vi "PSConverter.vi"(1 "Current States 2":string[][](table), 2 "PROC":string[](array[string]), 3 "STATES":string[][](array[string]), 4 "Input claster":cluster{u32, u8}[](array[cluster])) -> (0 "Current States":string[][](table))   [LabVIEW 2010]
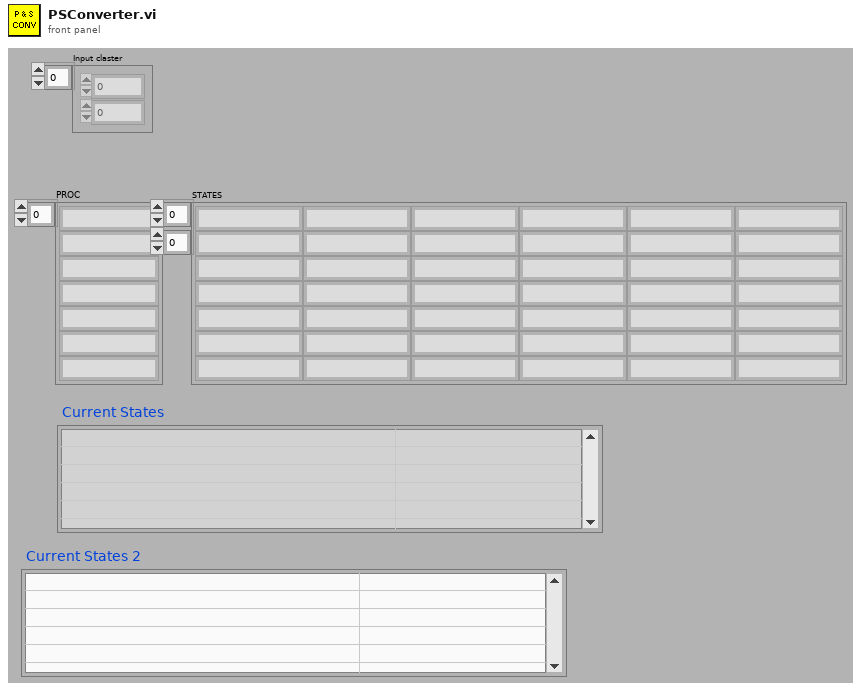
[diagram p1: front panel]
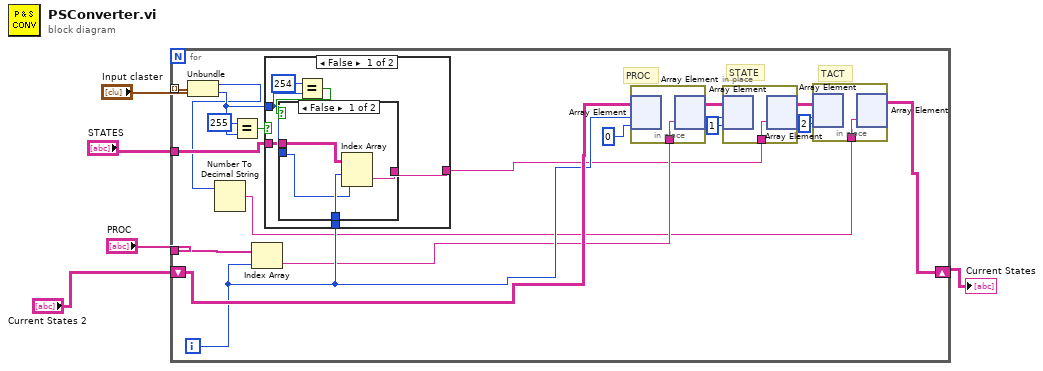
[diagram p0: block diagram]
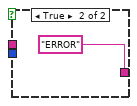
[diagram p2: hidden frame]
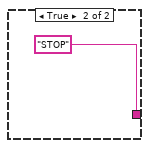
[diagram p3: hidden frame]
diagram:
  n1 = for {
    tunnel: "Input claster" -> [w25] mode=indexing
    tunnel: "PROC" -> [w21]
    tunnel: "STATES" -> [w20]
    shift-right: [w6] -> w5
    shift-left: "Current States 2" -> [w18]
    i -> [w17]
    # "TACT"
    # "STATE"
    # "PROC"
    n2 = Unbundle(w25) -> (w19:u32, w22:u8)
    n3 = Number To Decimal String(number=w19) -> (decimal integer string=w7:string)  [unwired: 1 in]
    n4 = Equal?(x=u8 255, y=w22) -> (x = y?=w23:bool)
    n5 = Index Array(array=w21, index=w17) -> (element=w15:string)
    n6 = case shown="False" w23 {
      tunnel: w22 -> [w31 _]
      tunnel: [w29 "STOP"] -> w8
      tunnel: w17 -> [w32 _]
      tunnel: w20 -> [w30 _]
      frame False {
        n7 = Equal?(x=u8 254, y=w31) -> (x = y?=w33:bool)
        n8 = case shown="False" w33 {
          tunnel: [w35 "ERROR"] -> w29
          tunnel: w32 -> [w38 _]
          tunnel: w31 -> [w37 _]
          tunnel: w30 -> [w36 _]
          frame False {
            n9 = Index Array(array=w36, index (row)=w38, index (col)=w37) -> (element=w35:string)
          }
          frame True {
          }
        }
      }
      frame True {
      }
    }
    n10 = in-place {
      in-place-border: w15 -> [w28]
      n11 = in-place-array #1(w18, w17, 0 ("disabled index (col)")) -> ()  [unwired: 1 out]
      n12 = in-place-array #1(w28) -> (w12:string[][], w14:i32)  [unwired: 1 out]
    }
    n13 = in-place {
      in-place-border: w8 -> [w27]
      n14 = in-place-array #2(w12, w14, 1) -> ()  [unwired: 1 out]
      n15 = in-place-array #2(w27) -> (w11:string[][], w13:i32)  [unwired: 1 out]
    }
    n16 = in-place {
      in-place-border: w7 -> [w26]
      n17 = in-place-array #3(w11, w13, 2) -> ()  [unwired: 1 out]
      n18 = in-place-array #3(w26) -> (w6:string[][])  [unwired: 2 out]
    }
  }
  "Current States" <- w5
